vi "Publisher Do.vi"(8 "error in (no error)":errorcluster, 10 "Publisher in":refnum<class "Publisher.lvclass">, 11 "Subscribe Msg":refnum<class "Publish Msg.lvclass">) -> (0 "error out":errorcluster, 2 "Publisher out":refnum<class "Publisher.lvclass">)   [LabVIEW 2020, in "Publisher.lvlib" / "Publish Msg.lvclass"]
doc: "This VI delivers the message to the actor by calling the appropriate method(s) on the actor."
uses:
  Publish Msg.lvclass
  C:/Current projects/WS/Framework/Framework/Actors/Publisher/Publisher Messages/Publisher Msg/Publisher Msg.lvclass
  Publisher/Publisher.lvclass
  Publisher Msg/Publisher Msg.lvclass/Publisher Msg.ctl
  Publish Msg.lvclass/Publish Msg.ctl
  PPL/HDH.Actor Framework.Core.Actor.lvlibp/1abvi3w/vi.lib/ActorFramework/Message/Message.lvclass
  Publisher Msg/Publisher Msg.lvclass
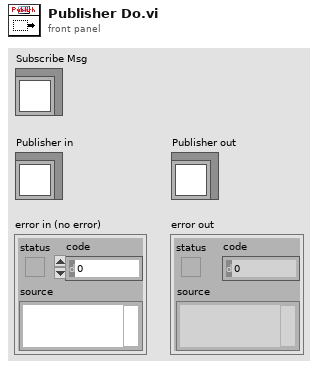
[diagram p1: front panel]
types:
  T1 = typedef "HDH.Actor Framework.Core.Actor.lvlibp/Message Enqueuer.lvclass/Message Priority.ctl" = enum16{"Low", "Normal", "High"}
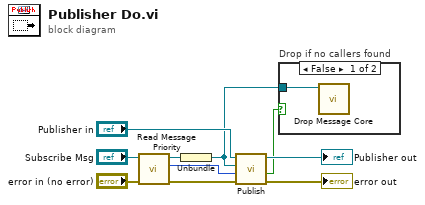
[diagram p0: block diagram]
diagram:
  n1 = call "Read Message Priority.vi"("error in (no error)"="error in (no error)", "Publisher Msg in"="Subscribe Msg") -> ("error out"=w4:errorcluster, "Message Priority"=w8:T1, "Publisher Msg out"=w9:refnum<class "Publish Msg.lvclass">)  [unwired: 7 in]
  n2 = Unbundle(w9) -> (w1:refnum<class "Message.lvclass">)
  n3 = call "Publish.vi"("error in (no error)"=w4, "Message Priority (Normal)"=w8, "Message"=w1, "Publisher in"="Publisher in") -> ("error out"=→"error out":errorcluster, "Callers found?"=w2:bool, "Publisher out"=→"Publisher out":refnum<class "Publisher.lvclass">)  [unwired: 5 in]
  n4 = case "Drop if no callers found" shown="False" w2 {
    tunnel: w1 -> [w11 _]
    frame False {
      n5 = call-dynamic "Drop Message Core.vi"("Message in"=w11) -> ()  [unwired: 11 in]
    }
    frame True {
    }
  }
